vi "Read Text.vi"(8 "error in (no error)":errorcluster, 9 "timeout ms (5000)":i32=5000, 11 "WebSocket in":refnum<class "WebSocket.lvclass">) -> (0 "error out":errorcluster, 2 "Data":string, 3 "WebSocket out":refnum<class "WebSocket.lvclass">)   [LabVIEW 2021, in "WebSockets.lvlib" / "WebSocket.lvclass"]
doc: "Reads a text frame from a WebSocket connection endpoint. Internally handles fragmented messages and Ping requests.\n\nIf a binary frame is received, the data will be returned and a warning generated.\nWebSockets 2.0.1.40\nSam Sharp - MediaMongrels Ltd\nCopyright (c) 2019, MediaMongrels Ltd"
uses:
  WebSocket.lvclass
  WebSocket.lvclass/WebSocket.ctl
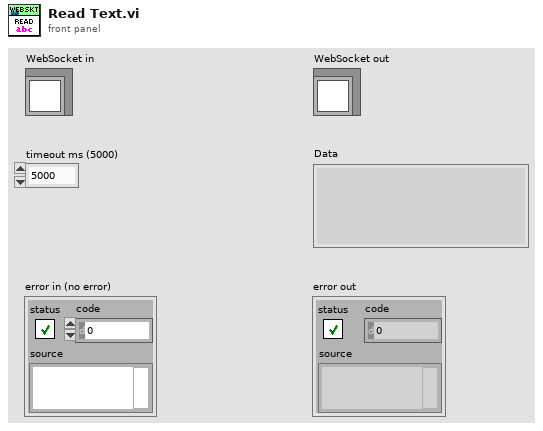
[diagram p1: front panel]
types:
  T1 = typedef "WebSockets.lvlib/WebSocket.lvclass/Opcodes.ctl" = u8
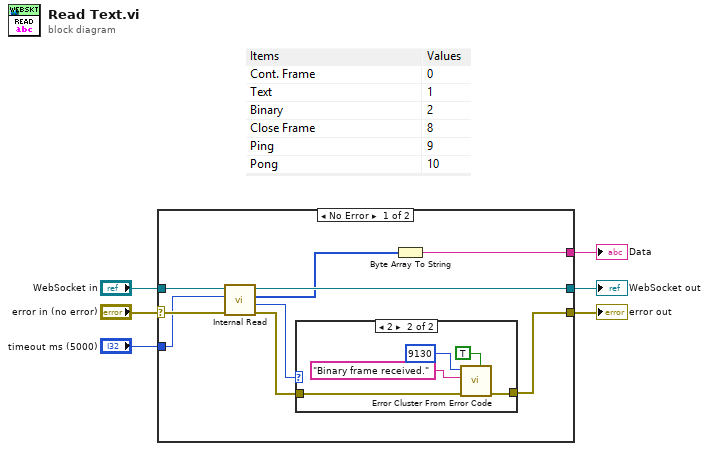
[diagram p0: block diagram]
diagram:
  n1 = case shown="No Error" "error in (no error)" {
    selector: "error in (no error)" -> [w14 w23]
    tunnel: [w10 w23] -> w5
    tunnel: [w11 w22] -> w3
    tunnel: "WebSocket in" -> [w15 w22]
    tunnel: "timeout ms (5000)" -> [w13 _]
    tunnel: [w9 _] -> w1
    frame No Error {
      n2 = call "Internal Read.vi"("error in (no error)"=w14, "timeout ms"=w13, "WebSocket in"=w15) -> ("error out"=w12:errorcluster, "Opcode"=w8:T1, "Data"=w7:u8[], "WebSocket out"=w11:refnum<class "WebSocket.lvclass">)  [unwired: 5 in]
      n3 = case shown="2" w8 {
        tunnel: w12 -> [w16 w21]
        tunnel: [w16 w17] -> w10
        frame Default {
        }
        frame 2 {
          n4 = call <vilib>:"Error Cluster From Error Code.vi"("is warning? (False)"=TRUE, "error in (no error)"=w21, "error message (\"\")"="Binary frame received." ("error message (\"\")"), "error code (0)"=9130) -> ("error out"=w17:errorcluster)  [unwired: 5 in]
        }
      }
      n5 = Byte Array To String(unsigned byte array=w7) -> (string=w9:string)
    }
    frame Error {
    }
  }
  "error out" <- w5
  "WebSocket out" <- w3
  "Data" <- w1
